vi "InitialStateNode_GetObjectStatus.vi"(0 "reference in":refnum<class "InitialStateNode.lvclass">, 5 "error in (no error)":errorcluster) -> (10 "All objects names":string[](array[string]), 12 "# of objects":i32, 13 "Class name":string, 14 "reference out":refnum<class "InitialStateNode.lvclass">, 15 "Not a refnum?":bool, 16 "Object name":string, 17 "All refs out":refnum<class "InitialStateNode.lvclass">[](array[class]), 18 "Attributes locked?":bool, 19 "error out":errorcluster)   [LabVIEW 2016, in "InitialStateNode.lvclass"]
doc: "Returns the object status and also information about all the objects in the class.\n\n[GOOP 2.0.15]"
uses:
  <resource>/Framework/Providers/Open_GDS/UML/InitialStateNode_class/InitialStateNode.lvclass
  <vilib>/addons/_goop3.llb/3GOOPStates.ctl
  <resource>/Framework/Providers/Open_GDS/UML/MultiLineString_class/MultiLineString.lvclass
panel:
  out "DebuggerOutput":string
  in  "DebuggerInput":string
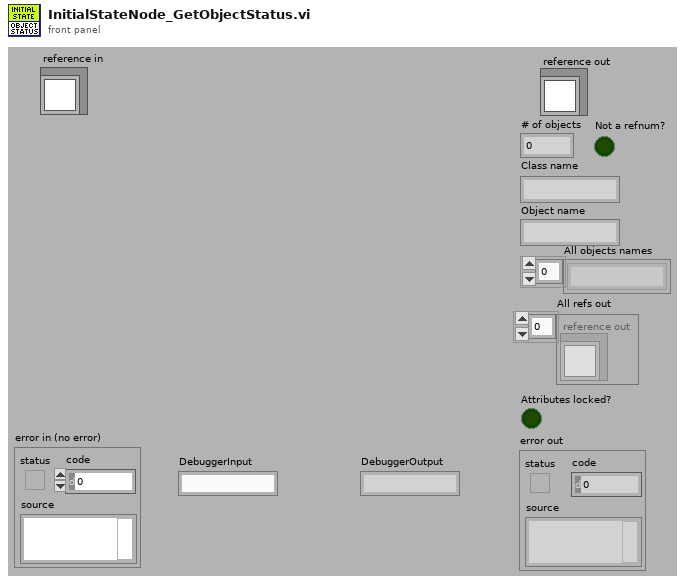
[diagram p1: front panel]
types:
  T1 = typedef "3GOOPStates.ctl" = enum16{"Set", "Get", "New", "Delete", "Clear", "Test and get", "Unlock data", "Information", "Look up existing", "New or look up existing", "Test and get shared", "Get shared", "Set shared", "Unlock shared", "Find dynamic method", "Register dynamic method", "Preload dynamic method", "Probe", "Cast to more generic", "Cast to more specific"}
  T2 = cluster{"Mode":enum16{"Get", "Set", "Delete"}, "Ref":i32, "ObjAttribute":string, "ClassAttribute":string}
  T3 = cluster{"Object names":string[], "Refs":i32[], "ObjectAttributeLocked":bool, "ClassAttributeLocked":bool, "ObjAttribute":variant, "ClassAttribute":variant}
  T4 = typedef "AbstractNode.lvclass/ObjectReference.ctl" = refnum<k1>
  T5 = typedef "3GOOPClassStatistics.ctl" = cluster{"# of waiting":u32, "Object names":string[], "Base class folders":path[], "Refs":i32[], "Class name":string}
  T6 = typedef "InitialStateNode.lvclass/ObjectAttributes.ctl" = cluster{"name":refnum<class "MultiLineString.lvclass">, "DEFAULT_WIDTH":i32, "DEFAULT_HEIGHT":i32}
  T7 = typedef "InitialStateNode.lvclass/ClassAttributes.ctl" = cluster{"Base class":T8, "childClassAttribute2":enum16{"Hello", "Goodbye"}}
  T8 = typedef "RectangularNode.lvclass/ClassAttributes.ctl" = cluster{"Base class":T9, "childClassAttribute2":enum16{"Hello", "Goodbye"}}
  T9 = typedef "AbstractNode.lvclass/ClassAttributes.ctl" = cluster{"classAttribute1":bool}
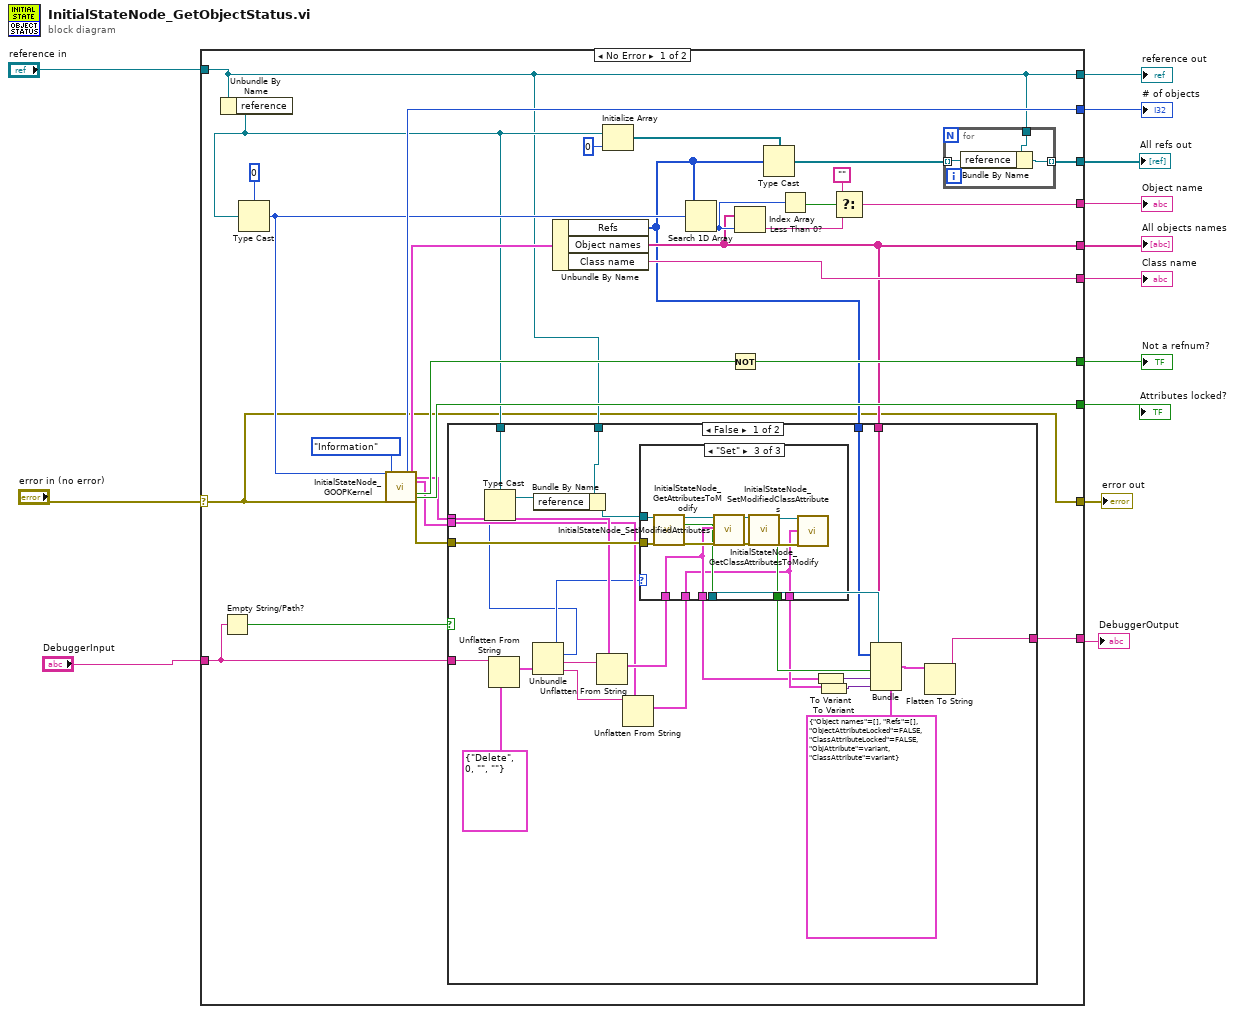
[diagram p0: block diagram]
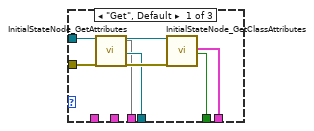
[diagram p2: hidden frame]
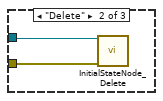
[diagram p3: hidden frame]
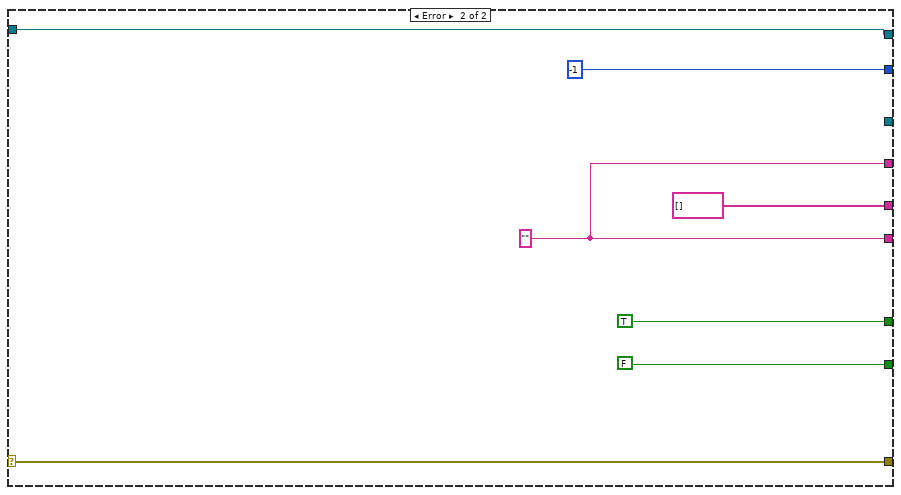
[diagram p5: hidden frame]
diagram:
  n1 = case shown="No Error" "error in (no error)" {
    selector: "error in (no error)" -> [w14 w101]
    tunnel: [w14 w101] -> w4
    tunnel: [w15 w95] -> w12
    tunnel: [w40 -1 ("# of objects")] -> w10
    tunnel: [w36 TRUE ("Exists?")] -> w7
    tunnel: [w37 FALSE] -> w8
    tunnel: [w35 w96] -> w1
    tunnel: [w20 string[] [] ("Object names")] -> w2
    tunnel: [w16 _] -> w11
    tunnel: [w29 w96] -> w3
    tunnel: "DebuggerInput" -> [w26 _]
    tunnel: [w18 _] -> w5
    tunnel: "reference in" -> [w15 w95]
    frame No Error {
      n2 = Unbundle By Name(w15) -> ("reference"=w21:T4)
      n3 = Empty String/Path?(string/path=w26) -> (empty?=w25:bool)
      n4 = Type Cast(type=0, x=w21) -> (*(type *) &x=w34:i32)
      n5 = call <resource>:"InitialStateNode_GOOPKernel.vi"("Ref in"=w34, "error in (no error)"=w14, "Action"=3GOOPStates."Information") -> ("# of objects"=w40:i32, "Class\nstatistics"=w38:T5, "Data out"=w24:T6, "Data shared out"=w23:T7, "Exists?"=w39:bool, "Data locked?"=w37:bool, "error out"=w22:errorcluster)  [unwired: 12 in, 6 out]
      n6 = Unbundle By Name(w38) -> ("Refs"=w19:i32[], "Object names"=w20:string[], "Class name"=w35:string)
      n7 = case shown="False" w25 {
        tunnel: w22 -> [w72 _]
        tunnel: w15 -> [w71 _]
        tunnel: w21 -> [w70 _]
        tunnel: [w63 _] -> w18
        tunnel: w24 -> [w58 _]
        tunnel: w23 -> [w57 _]
        tunnel: w26 -> [w55 _]
        tunnel: w19 -> [w52 _]
        tunnel: w20 -> [w51 _]
        frame False {
          n8 = Unflatten From String(type=T2 {"Mode"=enum."Delete", "Ref"=0, "ObjAttribute"="", "ClassAttribute"=""} ("DebuggerIn"), binary string=w55) -> (value=w60:T2)  [unwired: 1 in, 4 out]
          n9 = Unbundle(w60) -> ("Mode"=w56:enum16{"Get", "Set", "Delete"}, "Ref"=w53:i32, "ObjAttribute"=w61:string, "ClassAttribute"=w62:string)
          n10 = Type Cast(type=w70, x=w53) -> (*(type *) &x=w69:T4)
          n11 = Bundle By Name(cluster=w71, "reference"=w69) -> (w68:refnum<class "InitialStateNode.lvclass">)
          n12 = Unflatten From String(type=w58, binary string=w61) -> (value=w59:T6)  [unwired: 1 in, 4 out]
          n13 = Unflatten From String(type=w57, binary string=w62) -> (value=w54:T7)  [unwired: 1 in, 4 out]
          n14 = case shown="\"Set\"" w56 {
            tunnel: w72 -> [w80 w81 w93]
            tunnel: w68 -> [w79 w82 w94]
            tunnel: [w76 _ w85] -> w65
            tunnel: [w75 _ w84] -> w64
            tunnel: [w74 _ w86] -> w47
            tunnel: [w73 _ w83] -> w50
            tunnel: w59 -> [_ _ w86]
            tunnel: w54 -> [_ _ w83]
            frame "Get", Default {
              n15 = call <resource>:"InitialStateNode_GetAttributes.vi"("reference in"=w79, "error in (no error)"=w80) -> ("reference out"=w78:refnum<class "InitialStateNode.lvclass">, 16:w74, "DataRef"=w76:refnum<data-value>, "error out"=w77:errorcluster)  [unwired: 1 in, 13 out]
              n16 = call <resource>:"InitialStateNode_GetClassAttributes.vi"("reference in"=w78, "error in (no error)"=w77) -> ("Class attributes out"=w73:T7, "Attributes locked?"=w75:bool)  [unwired: 16 out]
            }
            frame "Delete" {
              n17 = call <resource>:"InitialStateNode_Delete.vi"("reference in"=w82, "error in (no error)"=w81) -> ()  [unwired: 18 out]
            }
            frame "Set" {
              n18 = call <resource>:"InitialStateNode_GetAttributesToModify.vi"("reference in"=w94, "error in (no error)"=w93) -> ("reference out"=w92:refnum<class "InitialStateNode.lvclass">, "Timeout"=w85:bool, "error out"=w91:errorcluster)  [unwired: 1 in, 14 out]
              n19 = call <resource>:"InitialStateNode_SetModifiedAttributes.vi"("reference in"=w92, "Attributes"=w86, "error in (no error)"=w91) -> ("reference out"=w90:refnum<class "InitialStateNode.lvclass">, "error out"=w89:errorcluster)  [unwired: 3 in, 12 out]
              n20 = call <resource>:"InitialStateNode_GetClassAttributesToModify.vi"("reference in"=w90, "error in (no error)"=w89) -> ("reference out"=w88:refnum<class "InitialStateNode.lvclass">, "Timeout"=w84:bool, "error out"=w87:errorcluster)  [unwired: 1 in, 14 out]
              n21 = call <resource>:"InitialStateNode_SetModifiedClassAttributes.vi"("reference in"=w88, "Class attributes"=w83, "error in (no error)"=w87) -> ()  [unwired: 2 in, 15 out]
            }
          }
          n22 = To Variant(anything=w47) -> (Variant=w48:variant)
          n23 = To Variant(anything=w50) -> (Variant=w49:variant)
          n24 = Bundle(cluster=T3 {"Object names"=[], "Refs"=[], "ObjectAttributeLocked"=FALSE, "ClassAttributeLocked"=FALSE, "ObjAttribute"=variant, "ClassAttribute"=variant}, "Object names"=w51, "Refs"=w52, "ObjectAttributeLocked"=w65, "ClassAttributeLocked"=w64, "ObjAttribute"=w48, "ClassAttribute"=w49) -> (w67:T3)
          n25 = Flatten To String(anything=w67) -> (data string=w63:string)  [unwired: 1 in, 4 out]
        }
        frame True {
        }
      }
      n26 = Initialize Array(w21, 0 ("Dimension Size")) -> (w27:T4[])
      n27 = Search 1D Array(1D array=w19, element=w34) -> (index of element=w33:i32)  [unwired: 1 out]
      n28 = Not(x=w39) -> (.not. x?=w36:bool)
      n29 = Index Array(array=w20, index=w33) -> (element=w31:string)
      n30 = Type Cast(type=w27, x=w19) -> (*(type *) &x=w17:T4[])
      n31 = Less Than 0?(x=w33) -> (x < 0?=w32:bool)
      n32 = Select(t="", s=w32, f=w31) -> (s? t:f=w29:string)
      n33 = for {
        tunnel: w17 -> [w45] mode=indexing
        tunnel: w15 -> [w44]
        tunnel: [w43] -> w16 mode=indexing
        n34 = Bundle By Name(cluster=w44, "reference"=w45) -> (w43:refnum<class "InitialStateNode.lvclass">)
      }
    }
    frame Error {
      w96 = "" ("Class name")
    }
  }
  "error out" <- w4
  "reference out" <- w12
  "# of objects" <- w10
  "Not a refnum?" <- w7
  "All refs out" <- w11
  "Attributes locked?" <- w8
  "Class name" <- w1
  "All objects names" <- w2
  "Object name" <- w3
  "DebuggerOutput" <- w5
